vi "Run device control.vi"() -> ()   [LabVIEW 2016]
uses:
  Device control.lvsc/Inputs.ctl
  Device control.lvsc
  Device control.lvsc/Outputs.ctl
  Device control.lvsc/Trigger.ctl
  <vilib>/Statechart/Infrastructure/RTStatechart/RunTime SCN.xnode
  Device control.lvsc/State.ctl
  Device control.lvsc/StatechartState.ctl
panel:
  out "Diagram Display":picture
  out "Active States":T1=[enum."NI.SC.Initial"]
  out "Outputs":T3
  out "Terminated?":bool
  in  "Diagram Display Index":u16
  in  "Trigger":T4
  in  "Inputs":T5 {"Status word" items=["Ready to switch on", "Switched on", "Operation enabled", "Fault", "Voltage enabled", "Quick stop", "Switch on disabled"]}
  in  "Init?":bool
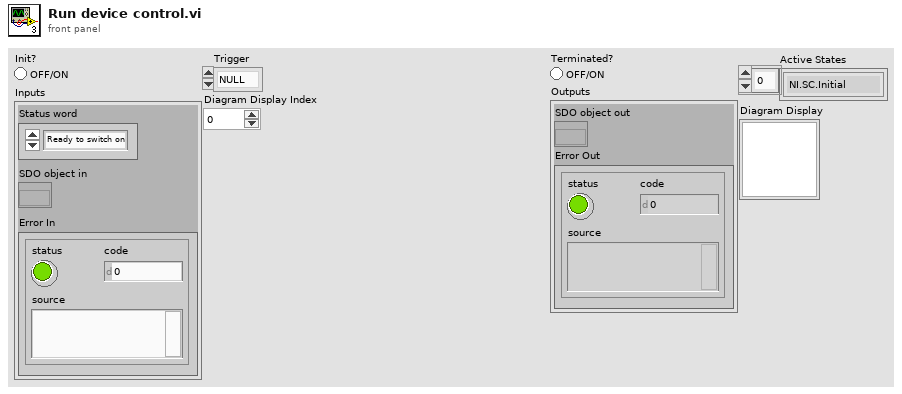
[diagram p1: front panel]
types:
  T1 = typedef "Device control.lvsc/StatechartState.ctl" = T2[]
  T2 = typedef "Device control.lvsc/State.ctl" = enum16{"NI.SC.Initial", "NI.SC.History", "NI.SC.ShallowHistory", "NI.SC.Terminal"}
  T3 = typedef "Device control.lvsc/Outputs.ctl" = cluster{"SDO object out":refnum<k20>, "Error Out":errorcluster}
  T4 = typedef "Device control.lvsc/Trigger.ctl" = enum16{"NULL", "Change state"}
  T5 = typedef "Device control.lvsc/Inputs.ctl" = cluster{"SDO object in":refnum<k20>, "Status word":u8, "Error In":errorcluster}
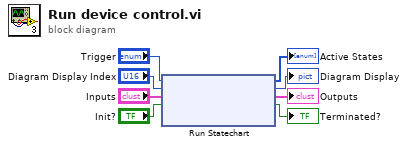
[diagram p0: block diagram]
diagram:
  n1 = xnode "Run Statechart"("Init?"="Init?", "Inputs"="Inputs", "Trigger"="Trigger", "Diagram Display Index"="Diagram Display Index") -> ("Terminated?"=→"Terminated?":bool, "Outputs"=→"Outputs":T3, "Active States"=→"Active States":T1, "Diagram Display"=→"Diagram Display":picture)
